vi "FPGA.vi"() -> ()   [LabVIEW 2018]
uses:
  PIC Select.ctl
  <vilib>/rvi/Emulation/niFpgaGetClockAttributes.vi
  <vilib>/rvi/Emulation/niFpgaSctlEmulationGetInTimedLoop.vi
  <vilib>/rvi/Emulation/niFpgaEmulationReportErrorSimple.vi
  <vilib>/rvi/eio/common/nirviEmuTemplateMethod_errors.vi
  <vilib>/rvi/Emulation/niFpgaCriticalErrorInLSC.vi
  <vilib>/eio/EIONode/EIONode.xnode
panel:
  in  "dsPIC33":T1=enum."Voltage"
  in  "Pause":u8
  in  "Delay":u16
  in  "Write":bool
  out "PIC Monitor":u64
  in  "Data":u64
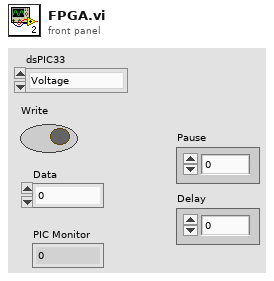
[diagram p1: front panel]
types:
  T1 = typedef "PIC Select.ctl" = enum16{"OFF", "Voltage", "Curtain", "Corona", "Heater"}
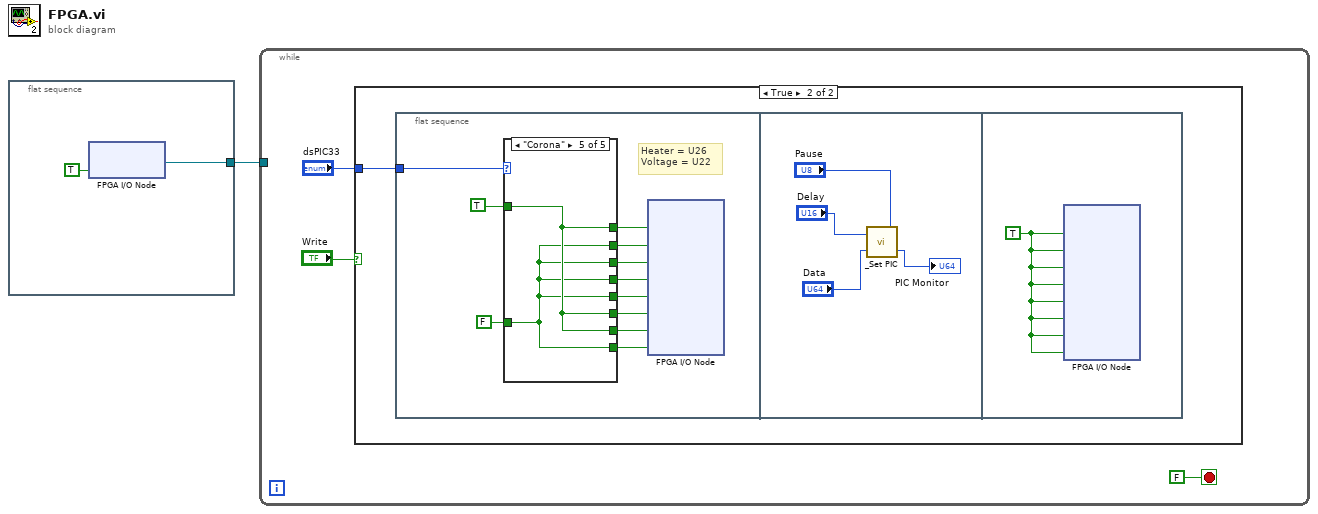
[diagram p0: block diagram]
diagram:
  n1 = flat-sequence {
    tunnel: [w2] -> w1
    frame #0 {
      n2 = xnode "FPGA I/O Node"("Elect"=TRUE) -> ("FPGA I/O Out"=w2:refnum<k21>)  [unwired: 1 in]
    }
  }
  n3 = while {
    tunnel: w1 -> [_]
    stop <- FALSE stop-if-true
    n4 = case shown="True" "Write" {
      tunnel: "dsPIC33" -> [_ w7]
      frame False {
      }
      frame True {
        n5 = flat-sequence {
          tunnel: w7 -> [w8]
          frame #0 {
            # "Heater = U26\nVoltage = U22"
            n6 = case shown="\"Corona\"" w8 {
              tunnel: TRUE -> [w19 w21 w23 w25 w27]
              tunnel: FALSE -> [_ w20 w22 w24 w26]
              tunnel: [w19 w20 w23 w24 w27] -> w16
              tunnel: [w19 w20 w22 w24 w26] -> w15
              tunnel: [w19 w20 w22 w24 w26] -> w14
              tunnel: [w19 w20 w22 w24 w26] -> w13
              tunnel: [w19 w21 w23 w24 w26] -> w12
              tunnel: [w19 w21 w23 w24 w26] -> w11
              tunnel: [w19 w20 w22 w25 w27] -> w10
              tunnel: [w19 w21 w23 w25 w27] -> w9
              frame "OFF", Default {
              }
              frame "Voltage" {
              }
              frame "Heater" {
              }
              frame "Curtain" {
              }
              frame "Corona" {
              }
            }
            n7 = xnode "FPGA I/O Node"("CS0"=w16, "CS1"=w14, "CS2"=w13, "BS0"=w12, "BS1"=w11, "BS2"=w10, "BS3"=w9, "BS3"=w15) -> ()  [unwired: 8 in, 8 out]
          }
          frame #1 {
            n8 = call "_Set PIC.vi"("Count(uSec)"="Pause", "Data"="Data", "Delay"="Delay") -> ("PIC Monitor"=→"PIC Monitor":u64)
          }
          frame #2 {
            w32 = TRUE
            n9 = xnode "FPGA I/O Node"("CS0"=w32, "CS1"=w32, "CS2"=w32, "BS0"=w32, "BS1"=w32, "BS2"=w32, "BS3"=w32, "BS3"=w32) -> ()  [unwired: 8 in, 8 out]
          }
        }
      }
    }
  }
